vi "Clear History.vi"(8 "Error In":errorcluster, 11 "BNT_XtGraph in":refnum<class "BNT_XtGraph.lvclass">) -> (0 "Error Out":errorcluster, 3 "BNT_XtGraph out":refnum<class "BNT_XtGraph.lvclass">)   [LabVIEW 2019, in "BNT_XtGraph.lvlib" / "BNT_XtGraph.lvclass"]
doc: "Clear history data."
uses:
  BNT_XtGraph.lvclass
  BNT_XtGraph.lvclass/BNT_XtGraph.ctl
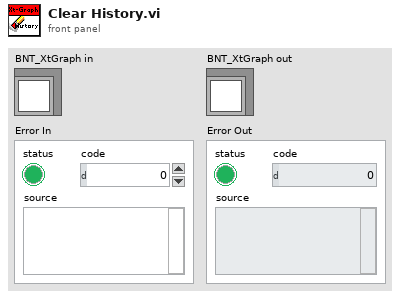
[diagram p1: front panel]
types:
  T1 = cluster{"X-t Value Pairs":cluster{"Time Stamp":timestamp, "Value":dbl}[]}[]
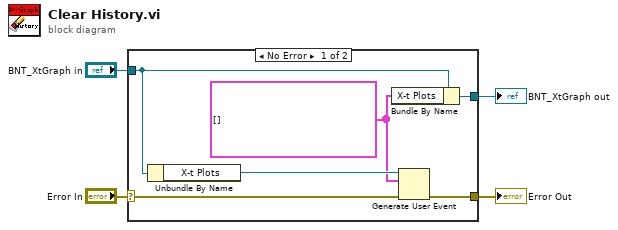
[diagram p0: block diagram]
diagram:
  n1 = case shown="No Error" "Error In" {
    selector: "Error In" -> [w6 w12]
    tunnel: [w5 w12] -> w2
    tunnel: [w10 w11] -> w3
    tunnel: "BNT_XtGraph in" -> [w9 w11]
    frame No Error {
      w7 = T1 [] ("X-t Plots")
      n2 = Unbundle By Name(w9) -> ("X-t Plots"=w8:refnum<user-event>)
      n3 = Bundle By Name(cluster=w9, "X-t Plots"=w7) -> (w10:refnum<class "BNT_XtGraph.lvclass">)
      n4 = Generate User Event(user event=w8, event data cluster=w7, error in=w6) -> (error out=w5:errorcluster)  [unwired: 1 in, 1 out]
    }
    frame Error {
    }
  }
  "BNT_XtGraph out" <- w3
  "Error Out" <- w2
